vi "GPS Aqq Module.vi"(7 "time zone":dbl, 8 "Error In":errorcluster, 11 "VISA resource name In":refnum<visa-resource-name>) -> (0 "Error Out":errorcluster, 1 "Status":string, 2 "Latitude [deg]":string, 3 "Longitude [deg]":string, 4 "Speed over ground [knots]":string, 5 "VISA resource name Out":refnum<visa-resource-name>)   [LabVIEW 2015]
panel:
  out "Time":string
  out "Mode":string
  out "Date [ddmmyy]":string
  out "Course over ground [degrees]":string
  out "E/W":string
  out "Longitude":string
  out "N/S":string
  out "Latitude":string
  out "UTC Time":string
  out "NMEA sentences":string
  # "GPS Aqq"
  # "[hhmmss.sss]"
  # "A = vAlid data\nV = inValid data"
  # "[ddmm.mmmm]"
  # "[dddmm.mmmm]"
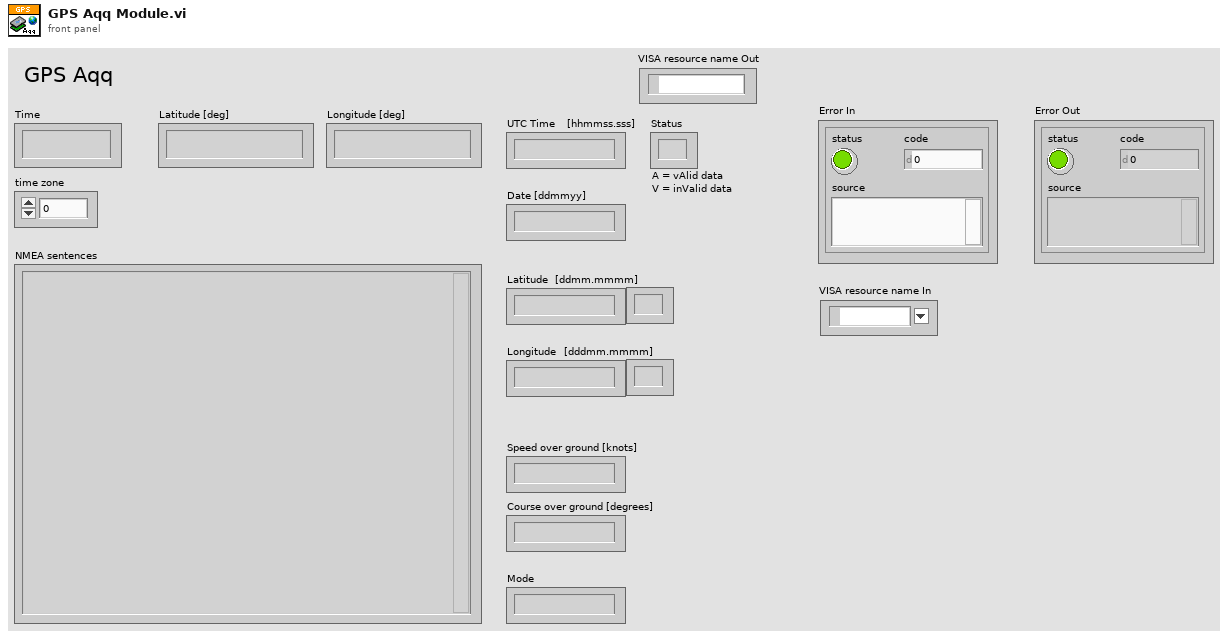
[diagram p1: front panel]
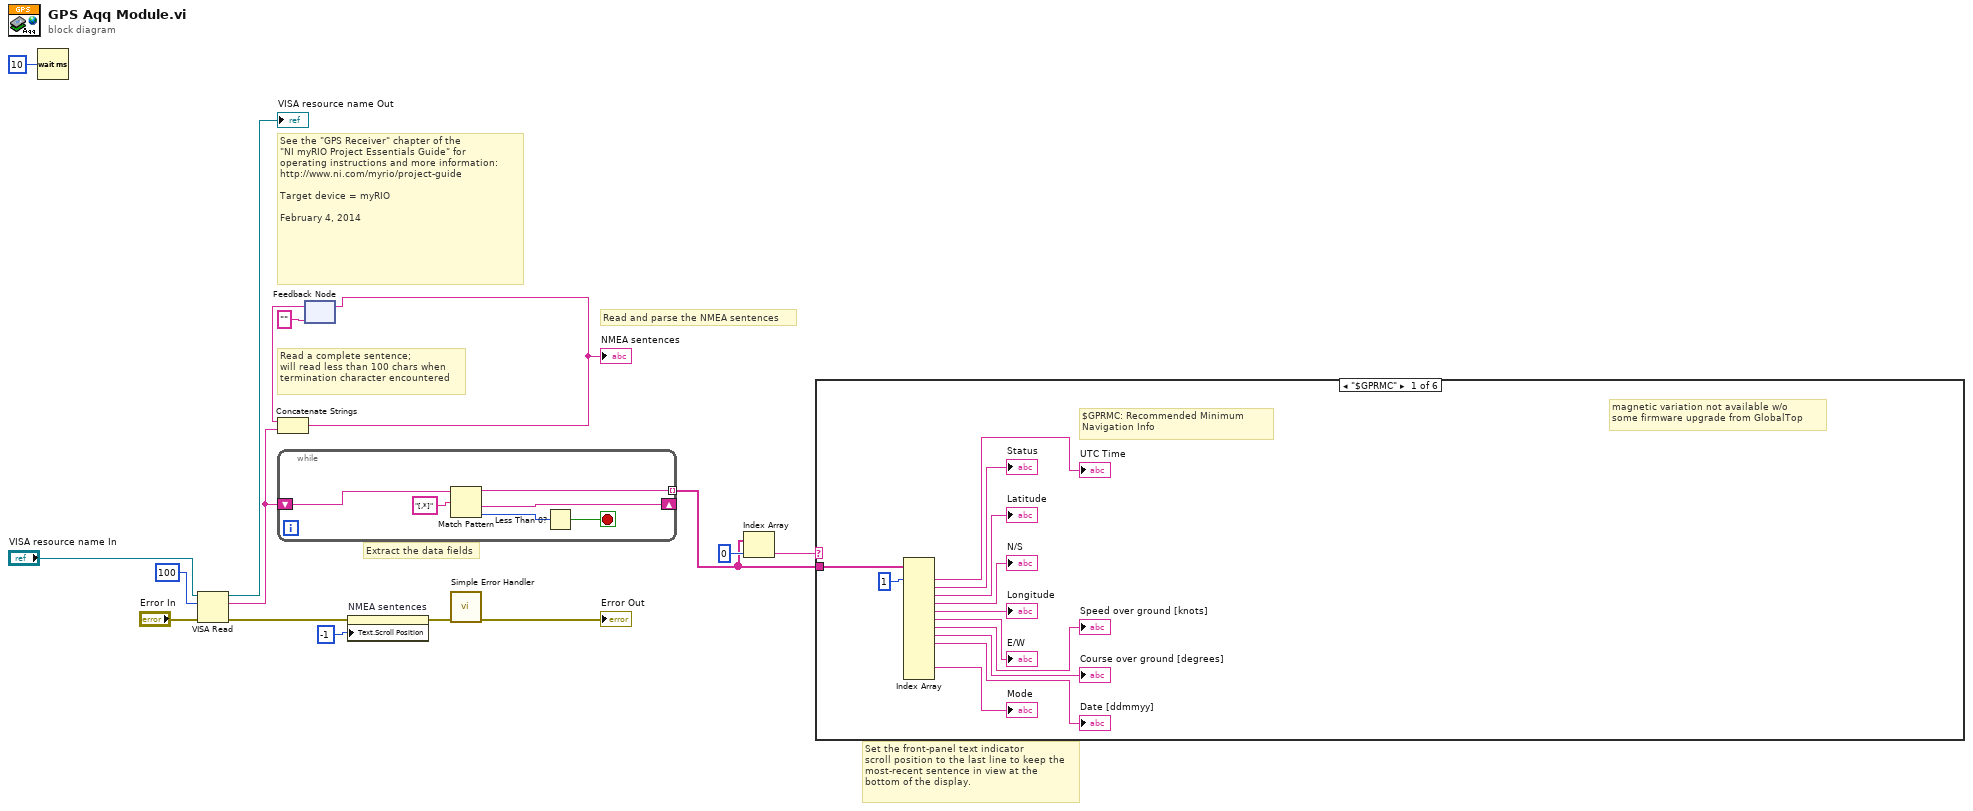
[diagram p0: block diagram]
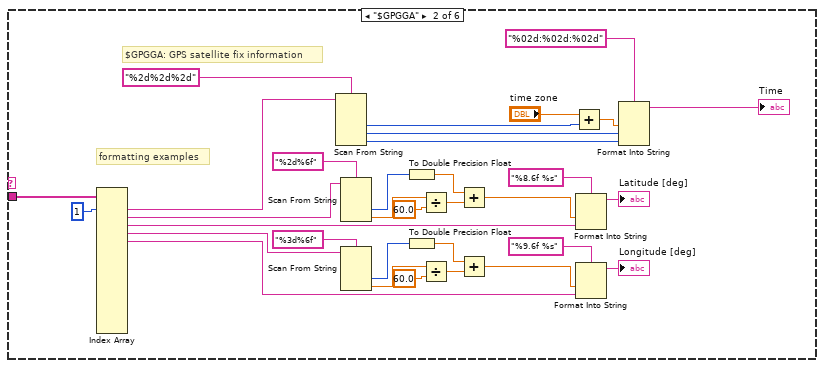
[diagram p2: hidden frame]
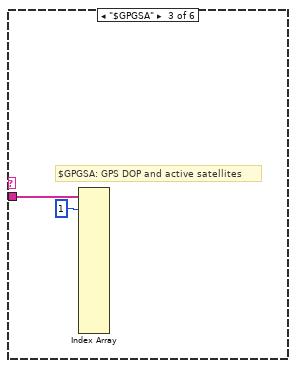
[diagram p3: hidden frame]
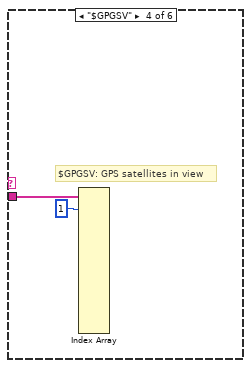
[diagram p4: hidden frame]
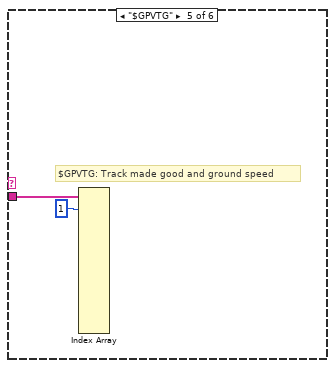
[diagram p5: hidden frame]
diagram:
  # "Extract the data fields"
  # "Set the front-panel text indicator\nscroll position to the last line to keep the\nmost-recent sentence in view at the\nbottom of the display."
  # "Read and parse the NMEA sentences"
  # "Read a complete sentence;\nwill read less than 100 chars when\ntermination character encountered"
  # "See the \"GPS Receiver\" chapter of the\n\"NI myRIO Project Essentials Guide\" for\noperating instructions and more information: \nhttp://www.ni.com/myrio/project-guide\n\nTarget device = myRIO\n\nFebruary 4, 2014"
  n1 = Wait (ms)(milliseconds to wait=u32 10) -> ()  [unwired: 1 out]
  n2 = VISA Read(VISA resource name="VISA resource name In", byte count=u32 100, error in (no error)="Error In") -> (VISA resource name out=→"VISA resource name Out":refnum<visa-resource-name>, read buffer=w10:string, error out=w15:errorcluster)  [unwired: 1 out]
  n3 = while {
    tunnel: [w20] -> w12 mode=indexing
    shift-right: [w19] -> _
    shift-left: w10 -> [w21]
    stop <- w18 stop-if-true
    n4 = Match Pattern(string=w21, regular expression="[,*]") -> (before substring=w20:string, after substring=w19:string, offset past match=w17:i32)  [unwired: 1 in, 1 out]
    n5 = Less Than 0?(x=w17) -> (x < 0?=w18:bool)
  }
  n6 = feedback #1("") -> (w8:string)
  n7 = Concatenate Strings "Concatenate Strings"(w8, w10) -> (w6:string)
  "NMEA sentences" <- w6
  n8 = feedback-in #1(w6) -> ()
  n9 = property on="NMEA sentences" class="Str"(error in=w15, "Text.Scroll Position"=-1) -> (error out=w4:errorcluster)  [unwired: 1 in, 1 out]
  n10 = call <vilib>:"Simple Error Handler.vi"("error in (no error)"=w4) -> ("error out"=→"Error Out":errorcluster)  [unwired: 4 in, 4 out]
  n11 = Index Array "Index Array"(array=w12, index=0) -> (element=w11:string)
  n12 = case shown="\"$GPRMC\"" w11 {
    tunnel: w12 -> [w34 w67 w69 w71 w73 _]
    frame "$GPRMC" {
      # "$GPRMC: Recommended Minimum\nNavigation Info"
      # "magnetic variation not available w/o\nsome firmware upgrade from GlobalTop"
      n13 = Index Array "Index Array"(array=w34, index #1=1 ("index")) -> (element #1=→"UTC Time":string, element #2=→"Status":string, element #3=→"Latitude":string, element #4=→"N/S":string, element #5=→"Longitude":string, element #6=→"E/W":string, element #7=→"Speed over ground [knots]":string, element #8=→"Course over ground [degrees]":string, element #9=→"Date [ddmmyy]":string, element #12=→"Mode":string)  [unwired: 12 in, 3 out]
    }
    frame "$GPGGA" {
      # "formatting examples"
      # "$GPGGA: GPS satellite fix information"
      n14 = Index Array "Index Array"(array=w67, index #1=1 ("index")) -> (element #1=w64:string, element #2=w55:string, element #3=w47:string, element #4=w36:string, element #5=w35:string)  [unwired: 15 in, 11 out]
      n15 = Scan From String "Scan From String"(format string="%2d%2d%2d", input string=w64) -> (output 1=w57:i32, output 2=w60:i32, output 3=w62:i32)  [unwired: 5 in, 3 out]
      n16 = Scan From String(format string="%2d%6f", input string=w55) -> (output 1=w52:i32, output 2=w54:dbl)  [unwired: 4 in, 3 out]
      n17 = Scan From String(format string="%3d%6f", input string=w36) -> (output 1=w40:i32, output 2=w38:dbl)  [unwired: 4 in, 3 out]
      n18 = To Double Precision Float(number=w52) -> (double precision float=w50:dbl)
      n19 = To Double Precision Float(number=w40) -> (double precision float=w42:dbl)
      n20 = Divide(x=w54, y=60.0) -> (x/y=w51:dbl)
      n21 = Divide(x=w38, y=60.0) -> (x/y=w41:dbl)
      n22 = Add(x=w50, y=w51) -> (x+y=w48:dbl)
      n23 = Add(x=w42, y=w41) -> (x+y=w44:dbl)
      n24 = Add(x="time zone", y=w57) -> (x+y=w58:dbl)
      n25 = Format Into String(format string="%8.6f %s", w48, w47) -> (resulting string=→"Latitude [deg]":string)  [unwired: 2 in, 1 out]
      n26 = Format Into String(format string="%9.6f %s", w44, w35) -> (resulting string=→"Longitude [deg]":string)  [unwired: 2 in, 1 out]
      n27 = Format Into String "Format Into String"(format string="%02d:%02d:%02d", w58, w60, w62) -> (resulting string=→"Time":string)  [unwired: 2 in, 1 out]
    }
    frame "$GPGSA" {
      # "$GPGSA: GPS DOP and active satellites"
      n28 = Index Array(array=w69, index #1=1 ("index")) -> ()  [unwired: 15 in, 16 out]
    }
    frame "$GPGSV" {
      # "$GPGSV: GPS satellites in view"
      n29 = Index Array(array=w71, index #1=1 ("index")) -> ()  [unwired: 15 in, 16 out]
    }
    frame "$GPVTG" {
      # "$GPVTG: Track made good and ground speed"
      n30 = Index Array(array=w73, index #1=1 ("index")) -> ()  [unwired: 15 in, 16 out]
    }
    frame Default {
    }
  }
